vi "Timeskip solution.vi"() -> ()   [LabVIEW 2015]
panel:
  in  "?":bool
  in  "?":bool
  in  "stop":bool
  out "A+B":dbl
  out "B":dbl
  out "A":dbl
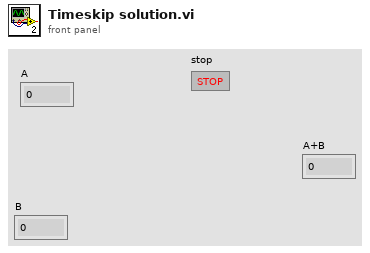
[diagram p1: front panel]
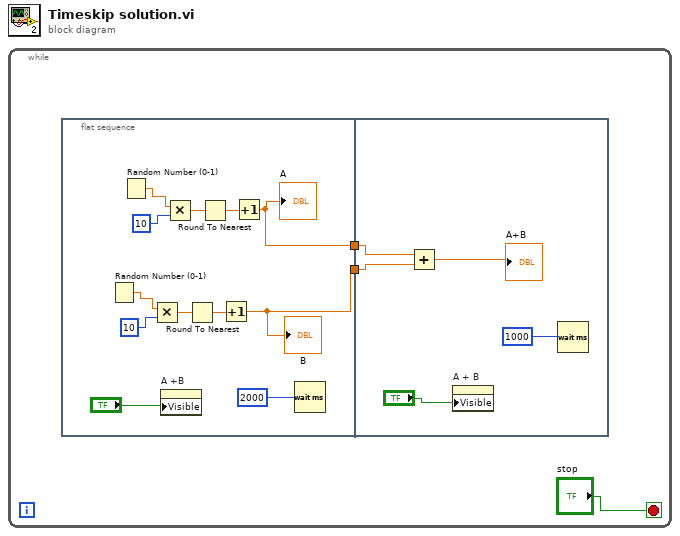
[diagram p0: block diagram]
diagram:
  n1 = while {
    stop <- "stop" stop-if-true
    n2 = flat-sequence {
      tunnel: [w11] -> w2
      tunnel: [w6] -> w1
      tunnel: w2 -> [w18]
      tunnel: w1 -> [w17]
      frame #0 {
        n3 = Random Number (0-1)() -> (number: 0 to 1=w10:dbl)
        n4 = Random Number (0-1)() -> (number: 0 to 1=w15:dbl)
        n5 = Multiply(x=w10, y=10) -> (x*y=w8:dbl)
        n6 = property on="A +B" class="Bool (strict)"("Visible"="?") -> ()  [unwired: 2 in, 2 out]
        n7 = Multiply(x=w15, y=10) -> (x*y=w13:dbl)
        n8 = Round To Nearest(number=w8) -> (nearest integer value=w7:dbl)
        n9 = Round To Nearest(number=w13) -> (nearest integer value=w12:dbl)
        n10 = Increment(x=w7) -> (x+1=w6:dbl)
        "B" <- w6
        n11 = Increment(x=w12) -> (x+1=w11:dbl)
        "A" <- w11
        n12 = Wait (ms)(milliseconds to wait=2000) -> ()  [unwired: 1 out]
      }
      frame #1 {
        n13 = Add(x=w18, y=w17) -> (x+y=→"A+B":dbl)
        n14 = property on="A + B" class="Bool (strict)"("Visible"="?") -> ()  [unwired: 2 in, 2 out]
        n15 = Wait (ms)(milliseconds to wait=1000) -> ()  [unwired: 1 out]
      }
    }
  }
